vi "Initialization.vi"(8 "error in (no error)":errorcluster, 10 "Setting":T1={"Termination"=1, "Baud Rate"=125000, "Interface"="CAN1", "XNET Database"="GIP_CAN_Database", "ECU"="GIP\nGIP_CAN_Database"} {"Termination" items=["Off", "On"]}, 11 "CAN in":refnum<class "CAN.lvclass">) -> (0 "error out":errorcluster, 3 "CAN out":refnum<class "CAN.lvclass">)   [LabVIEW 2019, in "CAN.lvclass"]
uses:
  CAN.lvclass
  Setting.ctl
  CAN.lvclass/CAN.ctl
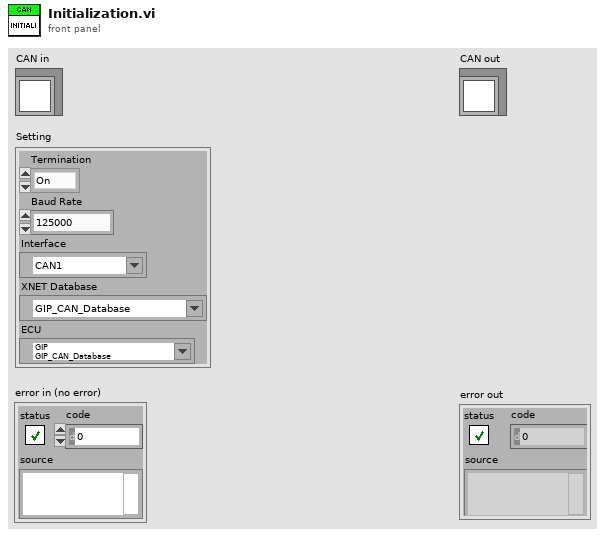
[diagram p1: front panel]
types:
  T1 = typedef "CAN.lvclass/Setting.ctl" = cluster{"Termination":u32, "Baud Rate":u64, "Interface":refnum<k21>, "XNET Database":refnum<k21>, "ECU":refnum<k21>}
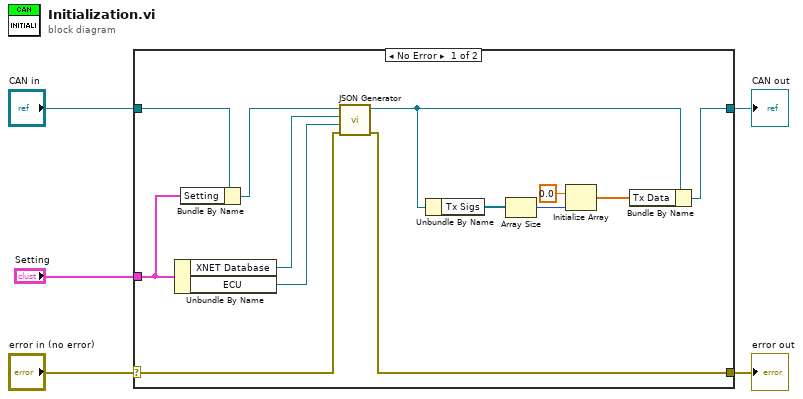
[diagram p0: block diagram]
diagram:
  n1 = case shown="No Error" "error in (no error)" {
    selector: "error in (no error)" -> [w18 w20]
    tunnel: [w17 w20] -> w4
    tunnel: [w12 w19] -> w2
    tunnel: "CAN in" -> [w8 w19]
    tunnel: "Setting" -> [w7 _]
    frame No Error {
      n2 = Unbundle By Name(w7) -> ("XNET Database"=w16:refnum<k21>, "ECU"=w15:refnum<k21>)
      n3 = Bundle By Name(cluster=w8, "Setting"=w7) -> (w6:refnum<class "CAN.lvclass">)
      n4 = call "JSON Generator.vi"("error in (no error)"=w18, "ECU"=w15, "XNET Database"=w16, "CAN in"=w6) -> ("error out"=w17:errorcluster, "CAN out"=w13:refnum<class "CAN.lvclass">)  [unwired: 6 in]
      n5 = Unbundle By Name(w13) -> ("Tx Sigs"=w14:refnum<k21>[])
      n6 = Array Size(array=w14) -> (size(s)=w11:i32)
      n7 = Initialize Array(0.0 ("element"), w11) -> (w9:dbl[])
      n8 = Bundle By Name(cluster=w13, "Tx Data"=w9) -> (w12:refnum<class "CAN.lvclass">)
    }
    frame Error {
    }
  }
  "error out" <- w4
  "CAN out" <- w2
